vi "populate sonde row cluster from sonde data cluster.vi"(5 "Final":bool, 7 "Initialize \nInitial Value \nCluster":bool, 8 "error in (no error)":errorcluster, 9 "Sonde Parameters \nInitial Values":T3 {"Salinity Initial" format="%_2f"; "Temp Initial" format="%_2f"; "ORP  Initial" format="%_2f"; "pH Initial" format="%_2f"; "DO Initial" format="%_2f"; "SC Initial" format="%_2f"}, 10 "Sample Sheet Data Row Cluster 2":T1 {"Cumulative\nVolume (ml)" format="%#_4g"; "Sonde Data Cluster"."Dissolved\nOxygen %" format="%_3g"; "Sonde Data Cluster"."Salinity" format="%_2g"; "Sonde Data Cluster"."Temp deg C" format="%_4g"; "Sonde Data Cluster"."ORP" format="%_4g"; "Sonde Data Cluster"."pH" format="%_4g"; "Sonde Data Cluster"."Dissolved\nOxygen mg/L" format="%_4g"; "Sonde Data Cluster"."Specific\nCond (uS)" format="%#_4g"}, 11 "Sonde Parameters \nTolerance Limits":T6 {"Salinity %" format="%_2f%%"; "Temp %" format="%_2f%%"; "ORP %" format="%_2f%%"; "pH %" format="%_2f%%"; "DO %" format="%_2f%%"; "SC %" format="%_2f%%"}) -> (0 "error out":errorcluster, 1 "Cluster":T4 {"Salinity"."%" format="%_2f%%"; "Salinity"."Value" format="%_4g"; "Temperature"."%" format="%_2f%%"; "Temperature"."Value" format="%_4g"; "ORP"."%" format="%_2f%%"; "ORP"."Value" format="%_4g"; "pH"."%" format="%_2f%%"; "pH"."Value" format="%_4g"; "Dissolved Oxygen"."%" format="%_2f%%"; "Dissolved Oxygen"."Value" format="%_4g"; "Sp. Cond. (uS/mL)"."%" format="%_2f%%"; "Sp. Cond. (uS/mL)"."Value" format="%_4g"; "Cumulative\nVolume" format="%#_4g"}, 6 "Sonde Parameters \nInitial Values Out":T3 {"Salinity Initial" format="%_2f"; "Temp Initial" format="%_2f"; "ORP  Initial" format="%_2f"; "pH Initial" format="%_2f"; "DO Initial" format="%_2f"; "SC Initial" format="%_2f"})   [LabVIEW 2016]
uses:
  activeXtest/activeXtest 2015 Folder/sonde cluster from excel.ctl
  Sonde Value Percent Tol.ctl
  activeXtest/activeXtest 2015 Folder/sample data row cluster.ctl
  activeXtest/activeXtest 2015 Folder/sonde cluster.ctl
panel:
  out "current time":timestamp
  in  "Input Cluster for % calculation":T4 caption="Cluster" {"Salinity"."%" format="%_2f%%"; "Salinity"."Value" format="%_4g"; "Temperature"."%" format="%_2f%%"; "Temperature"."Value" format="%_4g"; "ORP"."%" format="%_2f%%"; "ORP"."Value" format="%_4g"; "pH"."%" format="%_2f%%"; "pH"."Value" format="%_4g"; "Dissolved Oxygen"."%" format="%_2f%%"; "Dissolved Oxygen"."Value" format="%_4g"; "Sp. Cond. (uS/mL)"."%" format="%_2f%%"; "Sp. Cond. (uS/mL)"."Value" format="%_4g"; "Cumulative\nVolume" format="%#_4g"}
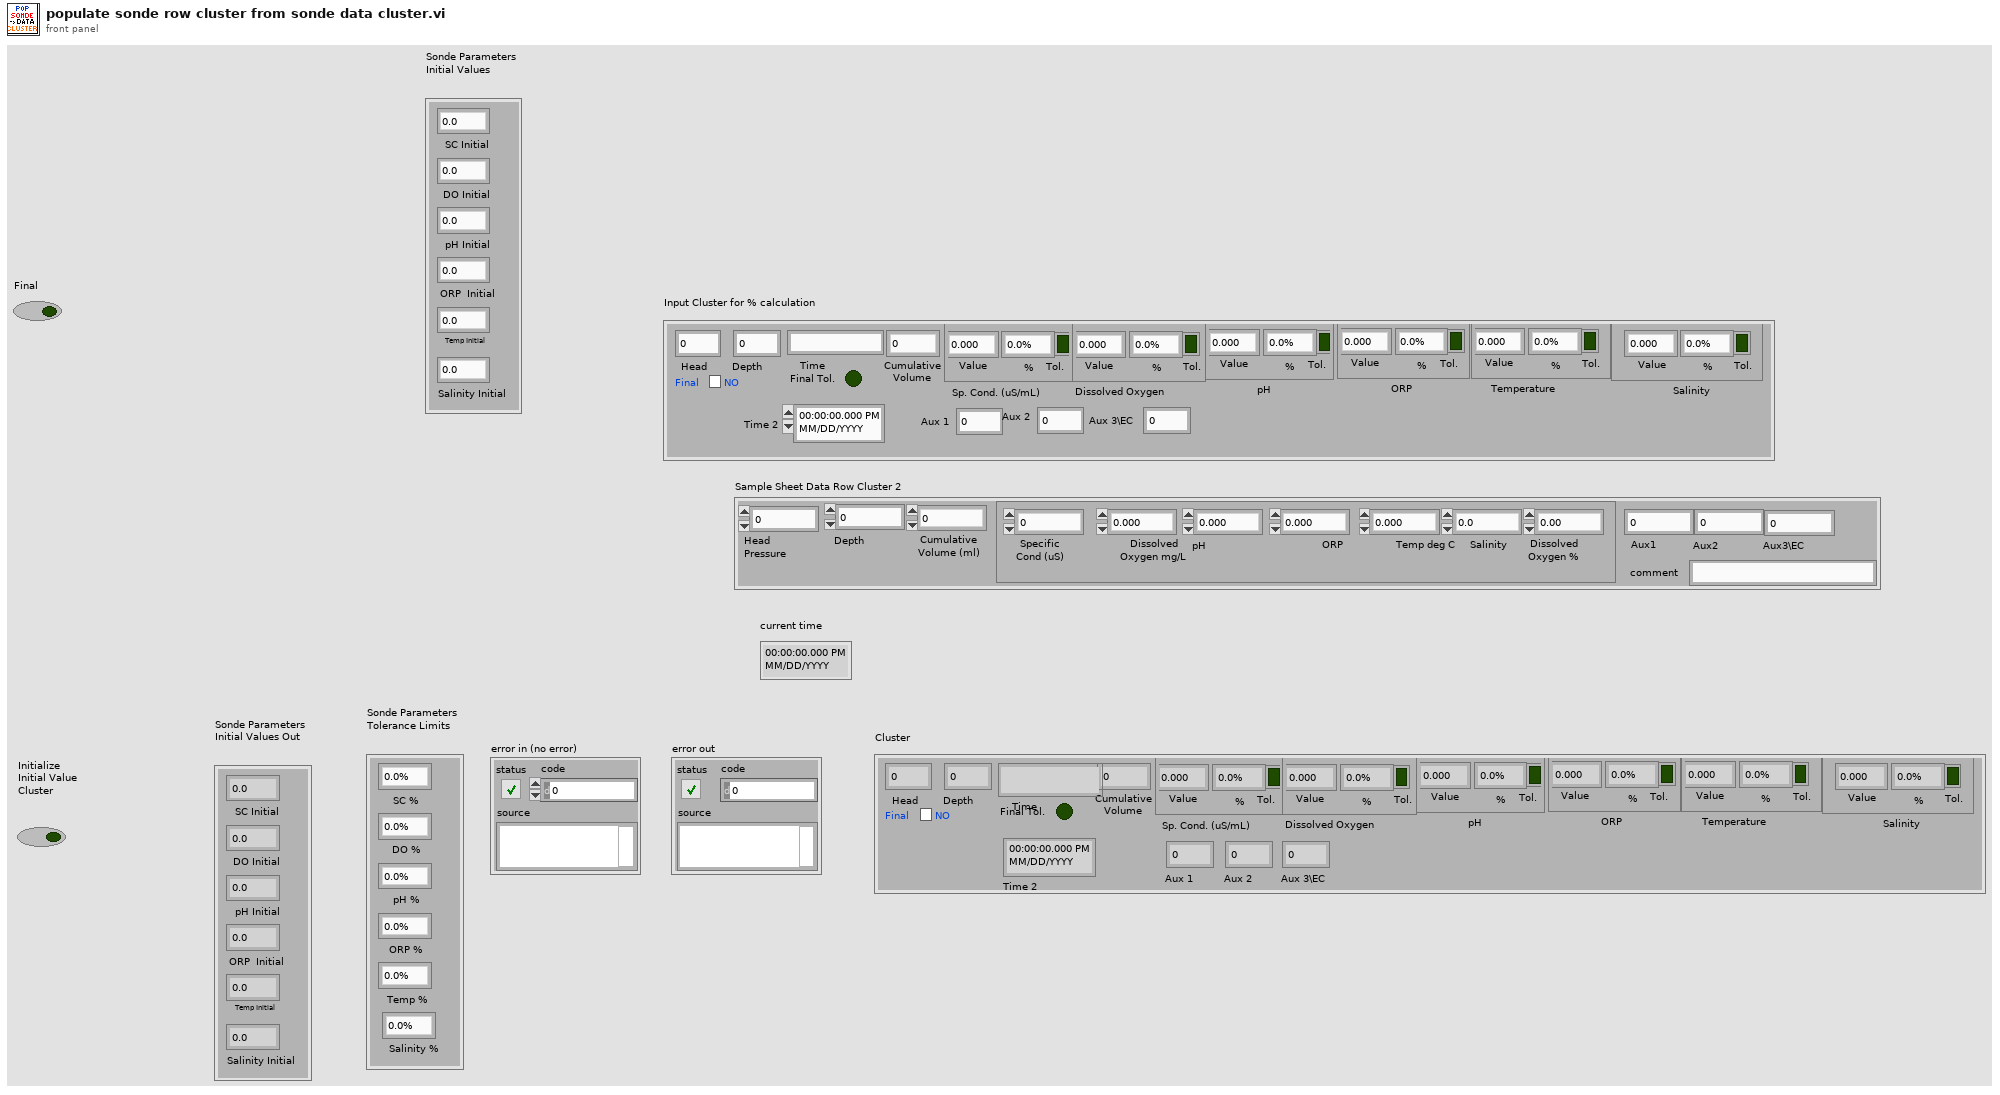
[diagram p1: front panel]
types:
  T1 = typedef "sample data row cluster.ctl" = cluster{"Head\nPressure":dbl, "Depth":dbl, "comment ":string, "Aux1":dbl, "Aux2":dbl, "Aux3\\EC":dbl, "Sonde Data Cluster":T2, "Cumulative\nVolume (ml)":dbl}
  T2 = typedef "sonde cluster.ctl" = cluster{"Specific\nCond (uS)":dbl, "Dissolved\nOxygen mg/L":dbl, "pH":dbl, "ORP":dbl, "Temp deg C":dbl, "Salinity":dbl, "Dissolved\nOxygen %":dbl}
  T3 = cluster{"SC Initial ":dbl, "DO Initial ":dbl, "pH Initial  ":dbl, "ORP  Initial":dbl, "Temp Initial":dbl, "Salinity Initial ":dbl}
  T4 = typedef "sonde cluster from excel.ctl" = cluster{"Head":dbl, "Depth":dbl, "Time":string, "Cumulative\nVolume":dbl, "Sp. Cond. (uS/mL)":T5, "Dissolved Oxygen":T5, "pH":T5, "ORP":T5, "Temperature":T5, "Salinity":T5, "Final Tol.":bool, "Final":bool, "Time 2":timestamp, "Aux 1":dbl, "Aux 2":dbl, "Aux 3\\EC":dbl}
  T5 = typedef "Sonde Value Percent Tol.ctl" = cluster{"Value":dbl, "%":dbl, "Tol.":bool}
  T6 = cluster{"SC %":dbl, "DO %":dbl, "pH % ":dbl, "ORP % ":dbl, "Temp % ":dbl, "Salinity %":dbl}
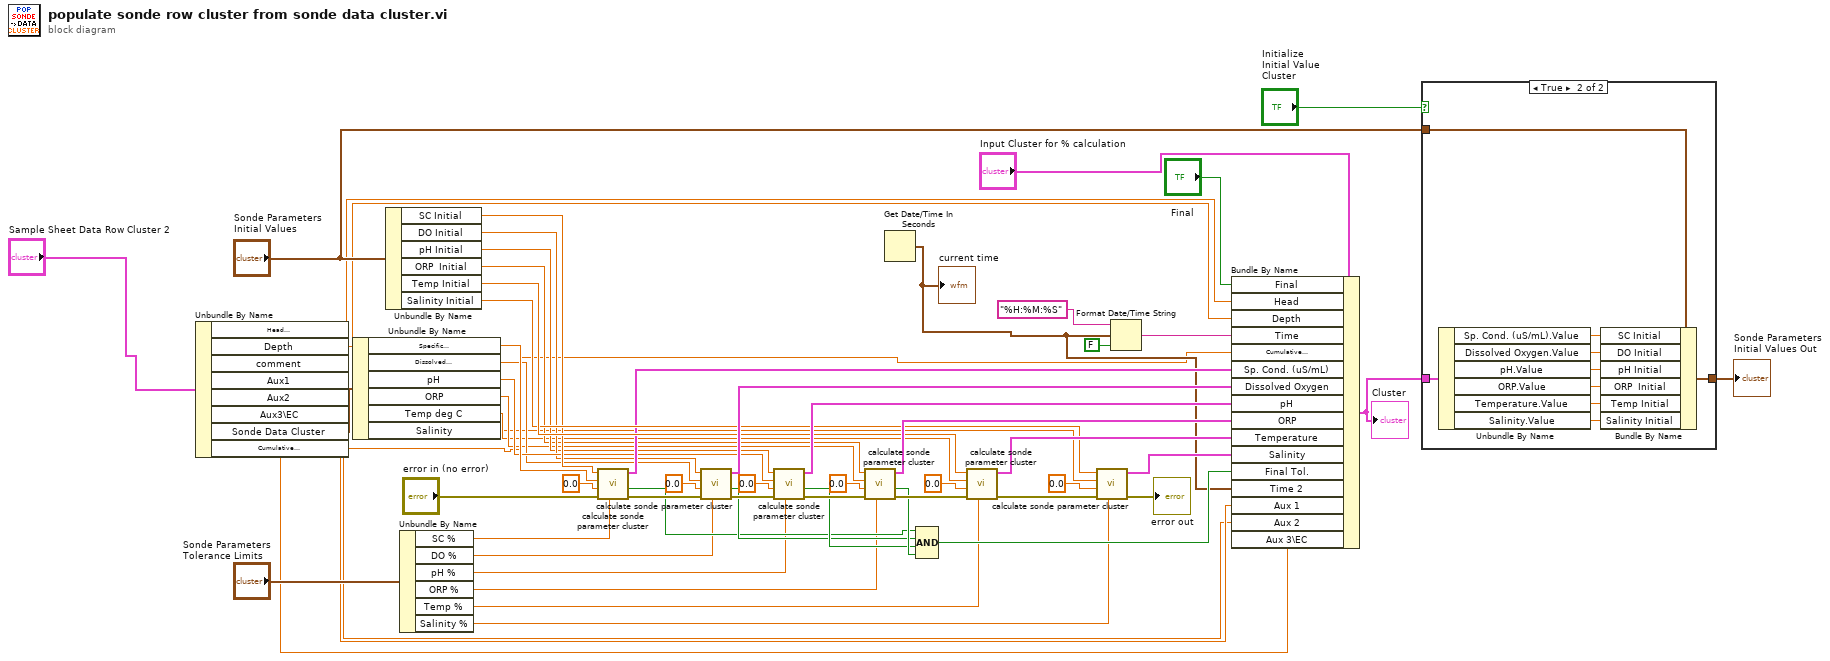
[diagram p0: block diagram]
diagram:
  n1 = Unbundle By Name("Sample Sheet Data Row Cluster 2") -> ("Head\nPressure"=w34:dbl, "Depth"=w33:dbl, "Aux1"=w6:dbl, "Aux2"=w5:dbl, "Aux3\\EC"=w4:dbl, "Sonde Data Cluster"=w2:T2, "Cumulative\nVolume (ml)"=w1:dbl)  [unwired: 1 out]
  n2 = Unbundle By Name(w2) -> ("Specific\nCond (uS)"=w28:dbl, "Dissolved\nOxygen mg/L"=w22:dbl, "pH"=w24:dbl, "ORP"=w15:dbl, "Temp deg C"=w12:dbl, "Salinity"=w10:dbl)
  n3 = Unbundle By Name("Sonde Parameters \nInitial Values") -> ("SC Initial"=w31:dbl, "DO Initial"=w20:dbl, "pH Initial"=w18:dbl, "ORP  Initial"=w16:dbl, "Temp Initial"=w39:dbl, "Salinity Initial"=w38:dbl)
  n4 = Unbundle By Name("Sonde Parameters \nTolerance Limits") -> ("SC %"=w30:dbl, "DO %"=w19:dbl, "pH %"=w23:dbl, "ORP %"=w14:dbl, "Temp %"=w43:dbl, "Salinity %"=w42:dbl)
  n5 = call "calculate sonde parameter cluster.vi"("tolerance limit"=w30, "error in (no error)"="error in (no error)", "Read % value"=0.0, "Read Value"=w28, "Initial Value"=w31) -> ("error out"=w27:errorcluster, "Tolerance"=w26:bool, "Cluster Out"=w29:T5)  [unwired: 3 in, 1 out]
  n6 = call "calculate sonde parameter cluster.vi"("tolerance limit"=w19, "error in (no error)"=w27, "Read % value"=0.0, "Read Value"=w22, "Initial Value"=w20) -> ("error out"=w60:errorcluster, "Tolerance"=w51:bool, "Cluster Out"=w46:T5)  [unwired: 3 in, 1 out]
  n7 = call "calculate sonde parameter cluster.vi"("tolerance limit"=w23, "error in (no error)"=w60, "Read % value"=0.0, "Read Value"=w24, "Initial Value"=w18) -> ("error out"=w59:errorcluster, "Tolerance"=w52:bool, "Cluster Out"=w47:T5)  [unwired: 3 in, 1 out]
  n8 = call "calculate sonde parameter cluster.vi"("tolerance limit"=w14, "error in (no error)"=w59, "Read % value"=0.0, "Read Value"=w15, "Initial Value"=w16) -> ("error out"=w58:errorcluster, "Tolerance"=w53:bool, "Cluster Out"=w48:T5)  [unwired: 3 in, 1 out]
  n9 = Get Date/Time In Seconds() -> (seconds since 1Jan1904=w7:timestamp)
  "current time" <- w7
  n10 = Compound Arithmetic op=AND(w26, w51, w52, w53) -> (w54:bool)
  n11 = call "calculate sonde parameter cluster.vi"("tolerance limit"=w43, "error in (no error)"=w58, "Read % value"=0.0, "Read Value"=w12, "Initial Value"=w39) -> ("error out"=w57:errorcluster, "Cluster Out"=w49:T5)  [unwired: 3 in, 2 out]
  n12 = call "calculate sonde parameter cluster.vi"("tolerance limit"=w42, "error in (no error)"=w57, "Read % value"=0.0, "Read Value"=w10, "Initial Value"=w38) -> ("error out"=→"error out":errorcluster, "Cluster Out"=w50:T5)  [unwired: 3 in, 2 out]
  n13 = Format Date/Time String(time format string (%c)="%H:%M:%S", seconds (now)=w7, UTC format=FALSE) -> (date/time string=w45:string)
  n14 = Bundle By Name(cluster="Input Cluster for % calculation", "Final"="Final", "Head"=w34, "Depth"=w33, "Time"=w45, "Cumulative\nVolume"=w1, "Sp. Cond. (uS/mL)"=w29, "Dissolved Oxygen"=w46, "pH"=w47, "ORP"=w48, "Temperature"=w49, "Salinity"=w50, "Final Tol."=w54, "Time 2"=w7, "Aux 1"=w6, "Aux 2"=w5, "Aux 3\\EC"=w4) -> (w35:T4)
  "Cluster" <- w35
  n15 = case shown="True" "Initialize \nInitial Value \nCluster" {
    tunnel: "Sonde Parameters \nInitial Values" -> [w62 w71]
    tunnel: [w62 w70] -> w37
    tunnel: w35 -> [_ w69]
    frame False {
    }
    frame True {
      n16 = Unbundle By Name(w69) -> ("Sp. Cond. (uS/mL).Value"=w68:dbl, "Dissolved Oxygen.Value"=w67:dbl, "pH.Value"=w66:dbl, "ORP.Value"=w65:dbl, "Temperature.Value"=w64:dbl, "Salinity.Value"=w63:dbl)
      n17 = Bundle By Name(cluster=w71, "SC Initial"=w68, "DO Initial"=w67, "pH Initial"=w66, "ORP  Initial"=w65, "Temp Initial"=w64, "Salinity Initial"=w63) -> (w70:T3)
    }
  }
  "Sonde Parameters \nInitial Values Out" <- w37
